vi "Write amplitude.vi"(8 "error in (no error)":errorcluster, 10 "amplitude":dbl=1.0, 11 "SignalIn in":refnum<class "SignalIn.lvclass">) -> (0 "error out":errorcluster, 3 "SignalIn out":refnum<class "SignalIn.lvclass">)   [LabVIEW 2011, in "SignalIn.lvclass"]
uses:
  SignalIn.lvclass
  SignalIn.lvclass/SignalIn.ctl
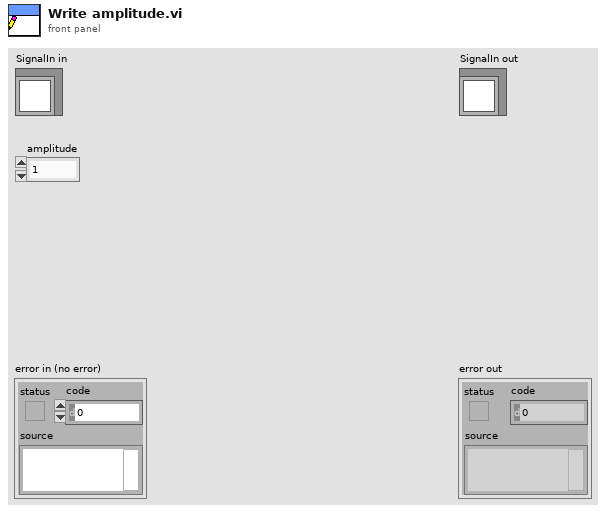
[diagram p1: front panel]
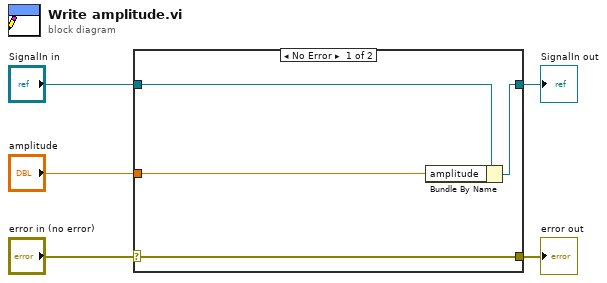
[diagram p0: block diagram]
diagram:
  n1 = case shown="No Error" "error in (no error)" {
    selector: "error in (no error)" -> [w9 w10]
    tunnel: [w9 w10] -> w4
    tunnel: [w7 w11] -> w2
    tunnel: "SignalIn in" -> [w8 w11]
    tunnel: "amplitude" -> [w6 _]
    frame No Error {
      n2 = Bundle By Name(cluster=w8, "amplitude"=w6) -> (w7:refnum<class "SignalIn.lvclass">)
    }
    frame Error {
    }
  }
  "error out" <- w4
  "SignalIn out" <- w2
